vi "Command Voltages Check.vi"() -> ()   [LabVIEW 2009]
uses:
  lib/Apps/On Off Button.ctl
  lib/Calibration/Command Voltage Check Ramp States.ctl
  Test Utilities/DAQ Read Actions.ctl
  <vilib>/DAQmx/write.llb/DAQmx Write (Analog 1D DBL NChan 1Samp).vi
  C:/Program Files (x86)/National Instruments/LabVIEW 2009/resource/objmgr/daqmx.rc
panel:
  out "Cmd Volt Chk Ramp States":T1
  in  "Ramping":T2
  in  "Number of\nIntervals":i32
  in  "Half Period (msec)":i32
  in  "Peak Value":dbl
  in  "Offset":dbl
  out "Diffs":dbl[](array[numeric])=[-7.680882880270997, -8.566659800159199, -9.658116593296763, -9.594949810916727, -8.940447035067507, -8.192445315897492] format="%^#_10g"
  out "Write error out":errorcluster
  out "Monitor":dbl[](array[numeric])=[-7.680882880270997, -8.566659800159199, -9.658116593296763, -9.594949810916727, -8.940447035067507, -8.192445315897492] format="%^#_10g"
  out "Command \nVoltage":dbl[](array[numeric])=[-0.0, -0.0, -0.0, -0.0, -0.0, -0.0] format="%^#_10g"
  out "Control Voltage":dbl[](array[numeric])=[-0.0, -0.0, -0.0, -0.0, -0.0, -0.0]
  in  "Quit":bool
  in  "rate":dbl=100.0
  in  "samples per \nchannel":i32=30 caption="samples per channel"
  in  "Command Voltage Task":refnum<k21>="Command Voltage"
  in  "Monitor Task":refnum<k21>="All Readings"
  in  "Actuator":i32(listbox)
  out "Command \nVoltages":T3(graph)={"Average[0]"=-7.17251209904047, "Average[1]"=-8.19396103384171, "Average[2]"=-9.68369051887908, "Average[3]"=-9.45574535938537, "Average[4]"=-9.241187346298316, "Average[5]"=-8.612741694704903, "Average[6]"=0.0, "Average[7]"=0.0, "Average[8]"=0.0}
  out "Monitor":T3(graph)={"Average[0]"=-7.17251209904047, "Average[1]"=-8.19396103384171, "Average[2]"=-9.68369051887908, "Average[3]"=-9.45574535938537, "Average[4]"=-9.241187346298316, "Average[5]"=-8.612741694704903, "Average[6]"=0.0, "Average[7]"=0.0, "Average[8]"=0.0}
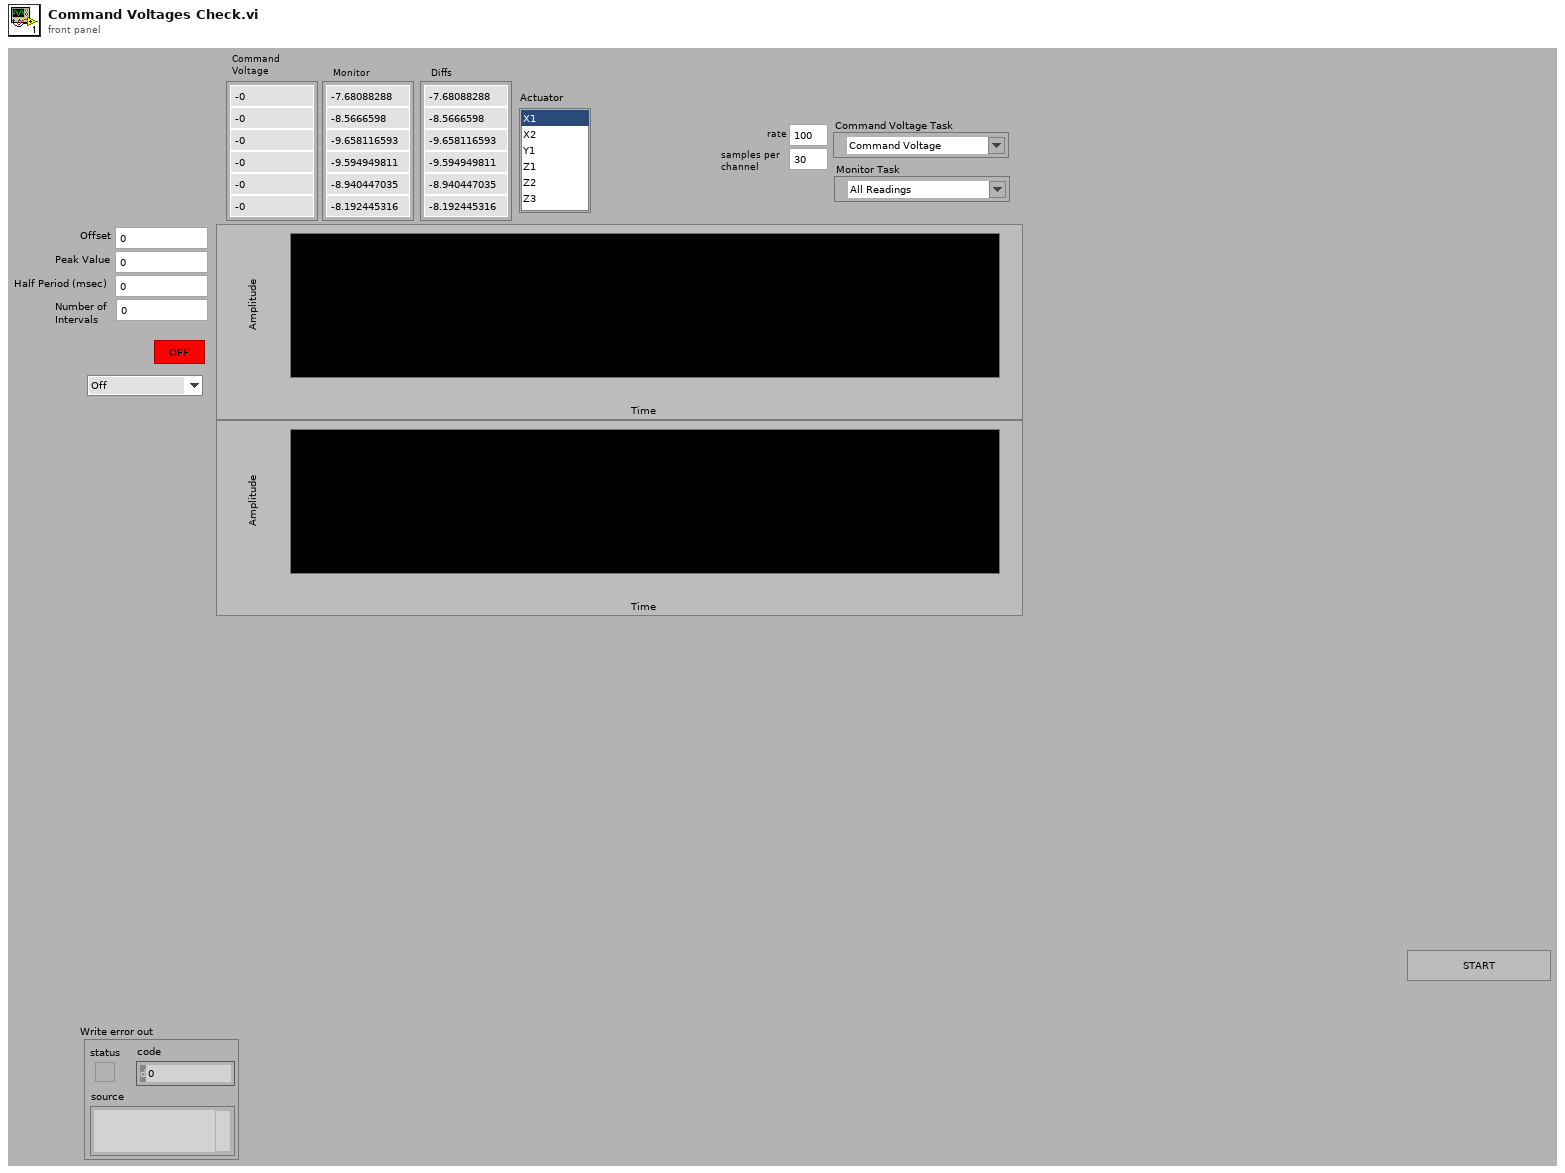
[diagram p1: front panel]
types:
  T1 = typedef "Command Voltage Check Ramp States.ctl" = enum16{"Off", "Start", "Ramp Up", "Ramp Down", "Stop"}
  T2 = typedef "On Off Button.ctl" = bool
  T3 = cluster{"Average[0]":dbl, "Average[1]":dbl, "Average[2]":dbl, "Average[3]":dbl, "Average[4]":dbl, "Average[5]":dbl, "Average[6]":dbl, "Average[7]":dbl, "Average[8]":dbl}
  T4 = typedef "DAQ Read Actions.ctl" = enum16{"Start", "Read", "Stop"}
  T5 = cluster{"Control Voltage[0]":dbl, "Control Voltage[1]":dbl, "Control Voltage[2]":dbl, "Control Voltage[3]":dbl, "Control Voltage[4]":dbl, "Control Voltage[5]":dbl, "Control Voltage[6]":dbl, "Control Voltage[7]":dbl, "Control Voltage[8]":dbl}
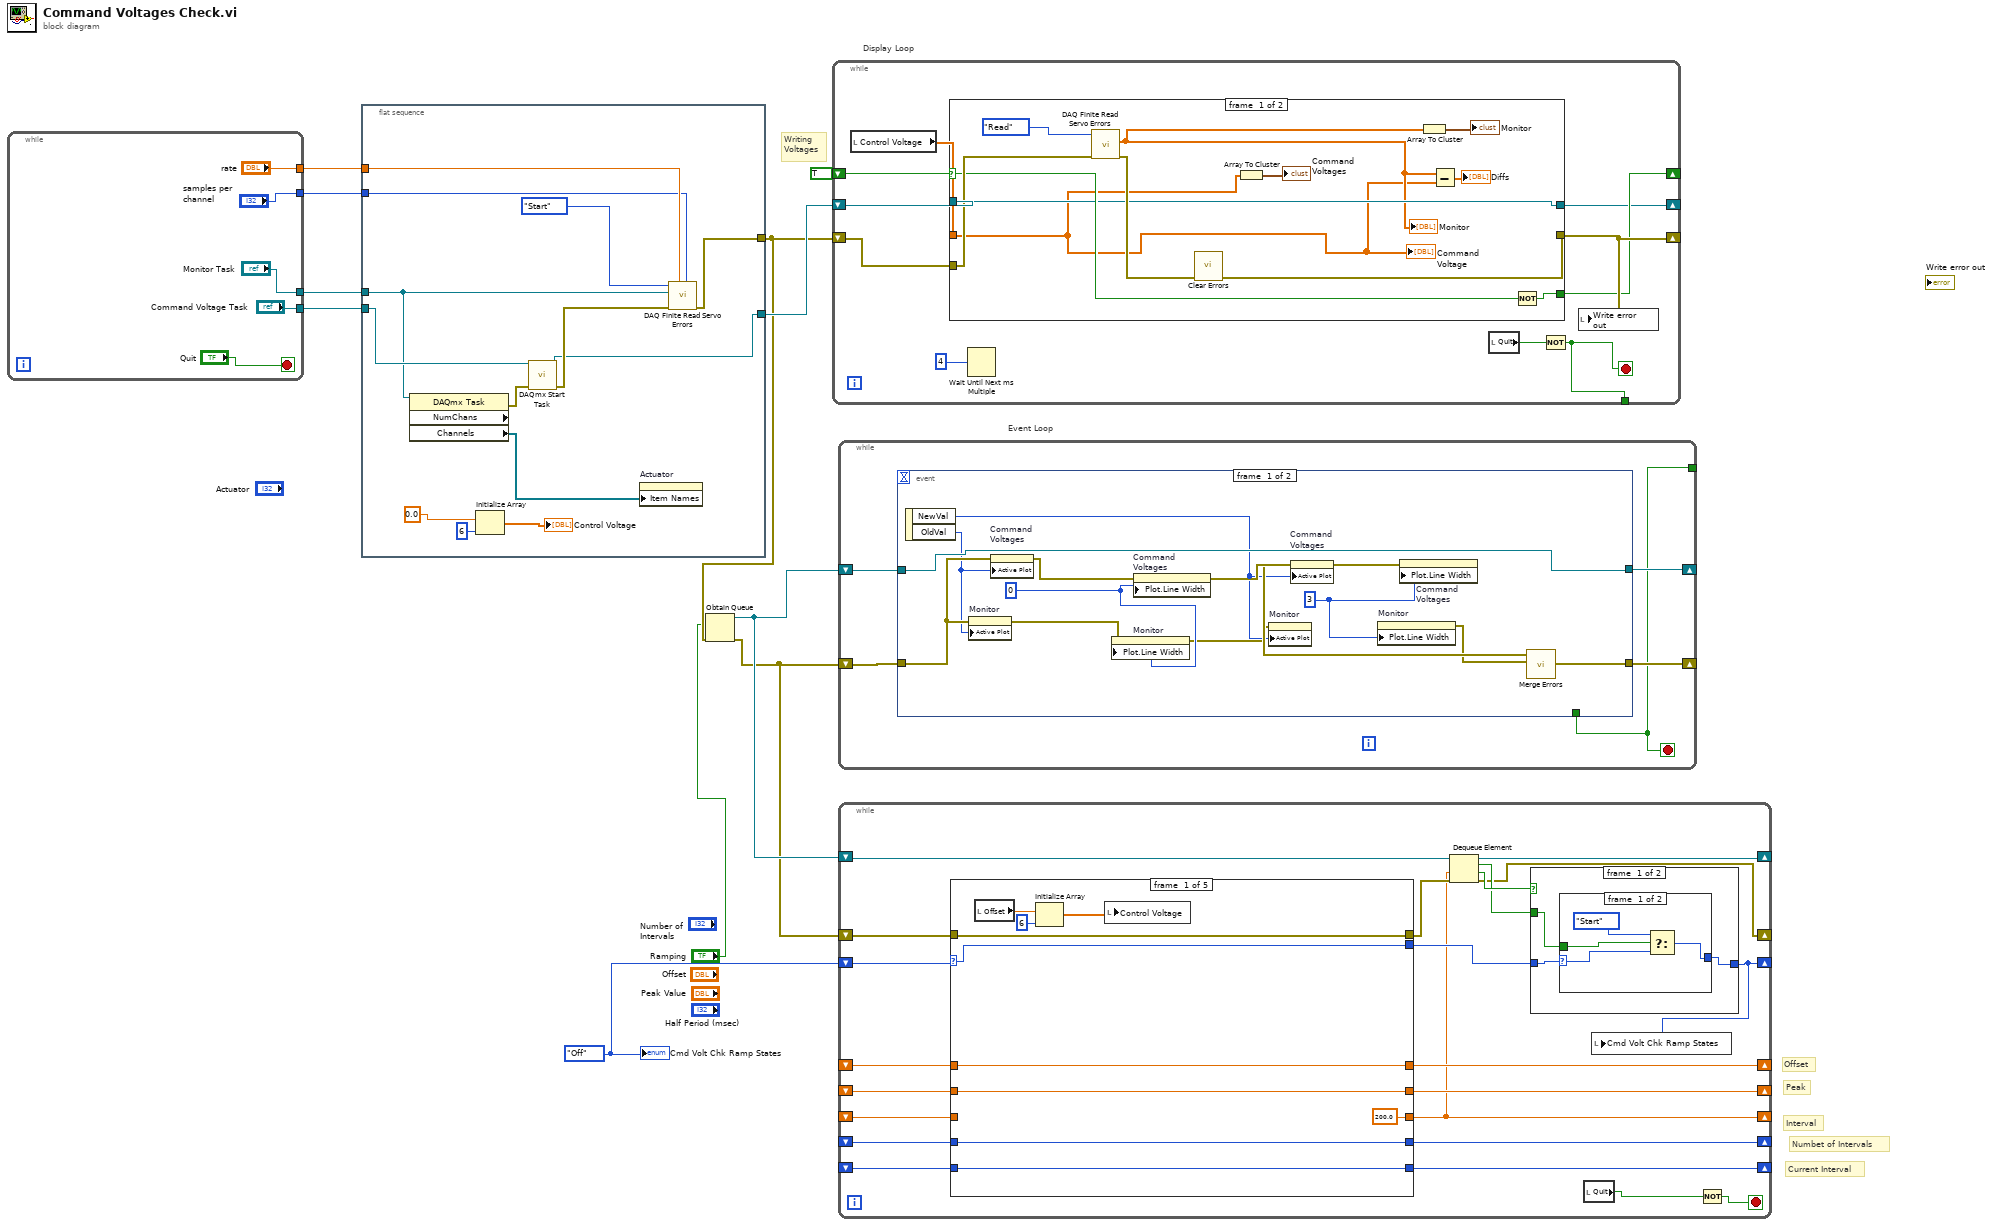
[diagram p0: block diagram]
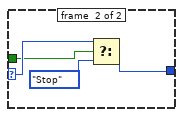
[diagram p2: hidden frame]
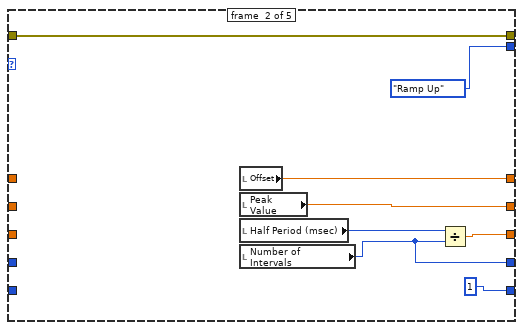
[diagram p4: hidden frame]
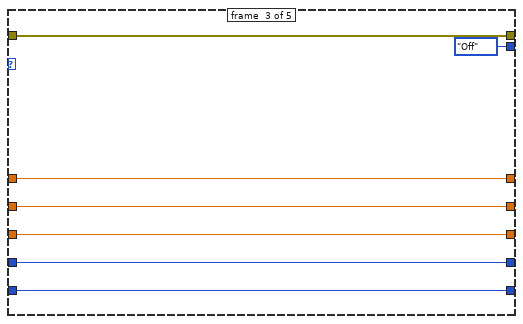
[diagram p5: hidden frame]
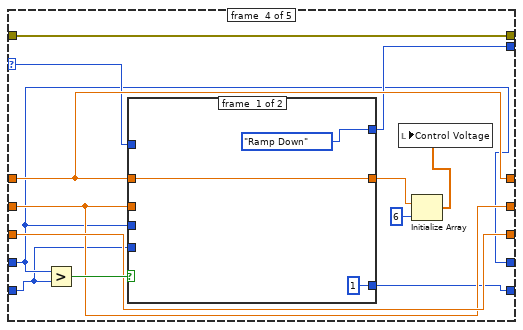
[diagram p6: hidden frame]
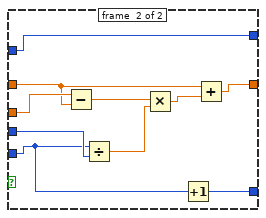
[diagram p7: hidden frame]
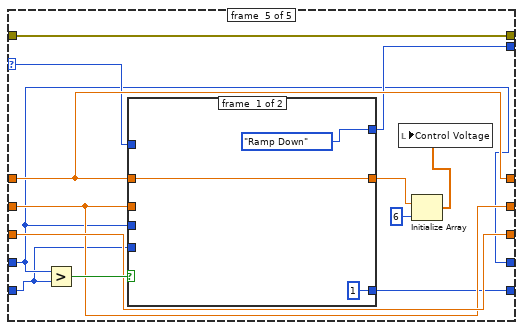
[diagram p8: hidden frame]
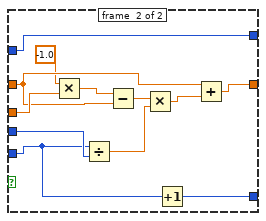
[diagram p9: hidden frame]
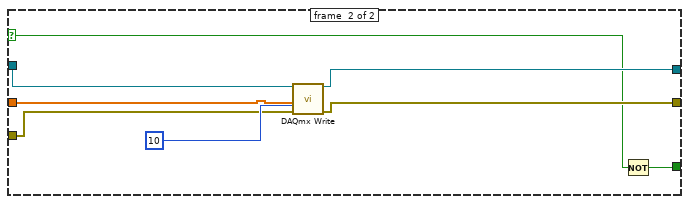
[diagram p10: hidden frame]
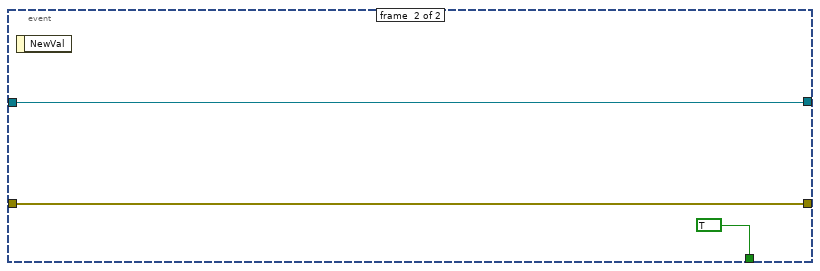
[diagram p11: hidden frame]
diagram:
  w5 = Command_Voltage_Check_Ramp_States."Off" ("Cmd Volt Chk Ramp States")
  # "Current Interval"
  # "Numbet of Intervals"
  # "Interval"
  # "Peak"
  # "Offset"
  # "Writing\nVoltages"
  n1 = while {
    tunnel: ["Command Voltage Task"] -> w11
    tunnel: ["Monitor Task"] -> w10
    tunnel: ["rate"] -> w9
    tunnel: ["samples per \nchannel"] -> w8
    stop <- "Quit" stop-if-true
  }
  n2 = flat-sequence {
    tunnel: w11 -> [w28]
    tunnel: w10 -> [w19]
    tunnel: w9 -> [w27]
    tunnel: w8 -> [w26]
    tunnel: [w21] -> w4
    tunnel: [w20] -> w7
    frame #0 {
      n3 = property class="DAQmx Task" props=["NumChans", "Channels"](reference=w19) -> (error out=w18:errorcluster, "Channels"=w17:refnum<k21>[])  [unwired: 1 in, 2 out]
      n4 = Initialize Array(0.0, 6 ("dimension size")) -> (→"Control Voltage":dbl[])
      n5 = call <vilib>:"DAQmx Start Task.vi"("task/channels in"=w28, "error in"=w18) -> ("task out"=w20:refnum<k21>, "error out"=w22:errorcluster)  [unwired: 12 out]
      n6 = property on="Actuator" class="LstBox (strict)"("Item Names"=w17) -> ()  [unwired: 2 in, 2 out]
      n7 = call "DAQ Finite Read Servo Errors.vi"("samples per channel"=w26, "rate"=w27, "error in"=w22, "task/channels in"=w19, "Action"=DAQ_Read_Actions."Start") -> ("error out"=w21:errorcluster)  [unwired: 6 out]
    }
  }
  n8 = Obtain Queue(element data type="Ramping", error in (no error)=w4) -> (queue out=w3:refnum<queue>, error out=w1:errorcluster)  [unwired: 3 in, 1 out]
  n9 = while "Display Loop" {
    shift-right: [w34] -> _
    shift-left: w4 -> [w35]
    tunnel: [w37] -> _
    shift-right: [w33] -> _
    shift-left: TRUE -> [w32]
    shift-right: [w30] -> _
    shift-left: w7 -> [w31]
    stop <- w37 stop-if-true
    n10 = local read "Control Voltage"() -> (w36:dbl[])
    n11 = case shown="False" w32 {
      selector: w32 -> [w45 w52]
      tunnel: w36 -> [w40 w55]
      tunnel: w35 -> [w48 w57]
      tunnel: [w46 w56] -> w34
      tunnel: [w44 w53] -> w33
      tunnel: w31 -> [w43 w58]
      tunnel: [w43 w54] -> w30
      frame #0 {
        n12 = call "DAQ Finite Read Servo Errors.vi"("error in"=w48, "Action"=DAQ_Read_Actions."Read") -> ("error out"=w47:errorcluster, "Average"=w41:dbl[])  [unwired: 3 in, 5 out]
        "Monitor" <- w41
        n13 = call <vilib>:"Clear Errors.vi"("error in (no error)"=w47) -> ("error out"=w46:errorcluster)  [unwired: 6 out]
        n14 = Array To Cluster(array=w40) -> (cluster=→"Command \nVoltages":T5)
        n15 = Array To Cluster(array=w41) -> (cluster=→"Monitor":T3)
        n16 = Subtract(x=w41, y=w40) -> (x-y=→"Diffs":dbl[])
        n17 = Not(x=w45) -> (.not. x?=w44:bool)
        "Command \nVoltage" <- w40
      }
      frame #1 {
        n18 = call-poly <vilib>:"DAQmx Write.vi"("task/channels in"=w58, "data"=w55, "timeout"=10, "error in"=w57) -> ("task out"=w54:refnum<k21>, "error out"=w56:errorcluster)  [unwired: 1 in, 9 out]
        n19 = Not(x=w52) -> (.not. x?=w53:bool)
      }
    }
    n20 = Wait Until Next ms Multiple(millisecond multiple=4) -> ()  [unwired: 1 out]
    n21 = local read "Quit"() -> (w38:bool)
    n22 = Not(x=w38) -> (.not. x?=w37:bool)
    n23 = local write "Write error out"(w34) -> ()
  }
  n24 = while "Event Loop" {
    tunnel: [w60] -> _
    shift-right: [w61] -> _
    shift-left: w1 -> [w63]
    shift-right: [w62] -> _
    shift-left: w3 -> [w64]
    stop <- w60 stop-if-true
    n25 = event shown="[1] \"Quit\": Value Change" {
      selector: _ -> [_ _]
      dyn-events: _ -> [_ _]
      timeout: _ -> [_ _]
      tunnel: w64 -> [w74 w79]
      tunnel: w63 -> [w73 w80]
      tunnel: [w74 w79] -> w62
      tunnel: [w66 w80] -> w61
      tunnel: [_ TRUE] -> w60
      event #0 {
        w67 = u8 3 ("Plot.Line Width")
        w71 = u8 0 ("Plot.Line Width")
        n26 = event-data() -> ("NewVal"=w68:i32, "OldVal"=w72:i32)  [unwired: 1 out]
        n27 = property on="Monitor" class="WFChart (strict)"(error in=w73, "Active Plot"=w72) -> (error out=w70:errorcluster)  [unwired: 1 in, 1 out]
        n28 = property on="Command \nVoltages" class="WFChart (strict)"(error in=w73, "Active Plot"=w72) -> (error out=w78:errorcluster)  [unwired: 1 in, 1 out]
        n29 = property on="Monitor" class="WFChart (strict)"(error in=w70, "Plot.Line Width"=w71) -> (error out=w69:errorcluster)  [unwired: 1 in, 1 out]
        n30 = property on="Command \nVoltages" class="WFChart (strict)"(error in=w78, "Plot.Line Width"=w71) -> (error out=w77:errorcluster)  [unwired: 1 in, 1 out]
        n31 = property on="Monitor" class="WFChart (strict)"(error in=w69, "Active Plot"=w68) -> ()  [unwired: 1 in, 2 out]
        n32 = property on="Command \nVoltages" class="WFChart (strict)"(error in=w77, "Active Plot"=w68) -> (error out=w76:errorcluster)  [unwired: 1 in, 1 out]
        n33 = property on="Monitor" class="WFChart (strict)"("Plot.Line Width"=w67) -> (error out=w65:errorcluster)  [unwired: 2 in, 1 out]
        n34 = property on="Command \nVoltages" class="WFChart (strict)"(error in=w76, "Plot.Line Width"=w67) -> (error out=w75:errorcluster)  [unwired: 1 in, 1 out]
        n35 = call <vilib>:"Merge Errors.vi"("error in 2 (no error)"=w65, "error in 1 (no error)"=w75) -> ("error out"=w66:errorcluster)  [unwired: 5 in]
      }
      event #1 {
        n36 = event-data() -> ()  [unwired: 2 out]
      }
    }
  }
  n37 = while {
    shift-right: [w85] -> _
    shift-left: w5 -> [w103]
    shift-right: [w96] -> _
    shift-left: w1 -> [w102]
    shift-right: [w95] -> _
    shift-left: w3 -> [w101]
    shift-right: [w84] -> _
    shift-left: _ -> [w88]
    shift-right: [w93] -> _
    shift-left: _ -> [w89]
    shift-right: [w94] -> _
    shift-left: _ -> [w90]
    shift-right: [w92] -> _
    shift-left: _ -> [w87]
    shift-right: [w91] -> _
    shift-left: _ -> [w86]
    stop <- w83 stop-if-true
    n38 = case shown="\"Stop\"" w103 {
      selector: w103 -> [w121 _ _ w145 w171]
      tunnel: w102 -> [w122 w126 w135 w153 w179]
      tunnel: [w122 w126 w135 w153 w179] -> w100
      tunnel: [w121 Command_Voltage_Check_Ramp_States."Ramp Up" ("Cmd Volt Chk Ramp States") Command_Voltage_Check_Ramp_States."Off" ("Cmd Volt Chk Ramp States") w144 w170] -> w97
      tunnel: [w120 w133 w140 w147 w173] -> w94
      tunnel: [w119 w132 w139 w146 w172] -> w93
      tunnel: [200.0 w130 w136 w151 w177] -> w84
      tunnel: [w117 w129 w138 w143 w169] -> w92
      tunnel: [w116 1 w137 w141 w167] -> w91
      tunnel: w90 -> [w120 _ w140 w147 w173]
      tunnel: w89 -> [w119 _ w139 w146 w172]
      tunnel: w88 -> [_ _ w136 w151 w177]
      tunnel: w87 -> [w117 _ w138 w143 w169]
      tunnel: w86 -> [w116 _ w137 w142 w168]
      frame #0 {
        n39 = local read "Offset"() -> (w125:dbl)
        n40 = Initialize Array(w125, 6 ("dimension size")) -> (w123:dbl[])
        n41 = local write "Control Voltage"(w123) -> ()
      }
      frame #1 {
        n42 = local read "Offset"() -> (w133:dbl)
        n43 = local read "Peak Value"() -> (w132:dbl)
        n44 = local read "Half Period (msec)"() -> (w131:i32)
        n45 = local read "Number of\nIntervals"() -> (w129:i32)
        n46 = Divide(x=w131, y=w129) -> (x/y=w130:dbl)
      }
      frame #2 {
      }
      frame #3 {
        n47 = Greater?(x=w143, y=w142) -> (0:w152:bool)
        n48 = case shown="False" w152 {
          tunnel: w146 -> [_ w162]
          tunnel: w147 -> [w156 w161]
          tunnel: [w156 w159] -> w149
          tunnel: w145 -> [_ w166]
          tunnel: [Command_Voltage_Check_Ramp_States."Ramp Down" ("Cmd Volt Chk Ramp States") w166] -> w144
          tunnel: w143 -> [_ w165]
          tunnel: w142 -> [_ w158]
          tunnel: [1 w157] -> w141
          frame #0 {
          }
          frame #1 {
            n49 = Subtract(x=w162, y=w161) -> (x-y=w164:dbl)
            n50 = Divide(x=w158, y=w165) -> (x/y=w163:dbl)
            n51 = Multiply(x=w164, y=w163) -> (x*y=w160:dbl)
            n52 = Increment(x=w158) -> (x+1=w157:i32)
            n53 = Add(x=w161, y=w160) -> (x+y=w159:dbl)
          }
        }
        n54 = Initialize Array(w149, 6 ("dimension size")) -> (w148:dbl[])
        n55 = local write "Control Voltage"(w148) -> ()
      }
      frame #4 {
        n56 = Greater?(x=w169, y=w168) -> (0:w178:bool)
        n57 = case shown="False" w178 {
          tunnel: w172 -> [_ w190]
          tunnel: w173 -> [w182 w189]
          tunnel: [w182 w187] -> w175
          tunnel: w171 -> [_ w194]
          tunnel: [Command_Voltage_Check_Ramp_States."Ramp Down" ("Cmd Volt Chk Ramp States") w194] -> w170
          tunnel: w169 -> [_ w193]
          tunnel: w168 -> [_ w184]
          tunnel: [1 w183] -> w167
          frame #0 {
          }
          frame #1 {
            n58 = Multiply(x=-1.0, y=w190) -> (x*y=w186:dbl)
            n59 = Divide(x=w184, y=w193) -> (x/y=w191:dbl)
            n60 = Subtract(x=w186, y=w189) -> (x-y=w192:dbl)
            n61 = Multiply(x=w192, y=w191) -> (x*y=w188:dbl)
            n62 = Increment(x=w184) -> (x+1=w183:i32)
            n63 = Add(x=w189, y=w188) -> (x+y=w187:dbl)
          }
        }
        n64 = Initialize Array(w175, 6 ("dimension size")) -> (w174:dbl[])
        n65 = local write "Control Voltage"(w174) -> ()
      }
    }
    n66 = Dequeue Element(queue=w101, timeout in ms (-1)=w84, error in (no error)=w100) -> (queue out=w95:refnum<queue>, element=w98:T2, timed out?=w99:bool, error out=w96:errorcluster)
    n67 = case shown="False" w99 {
      tunnel: w98 -> [w105 _]
      tunnel: w97 -> [w106 w115]
      tunnel: [w104 w115] -> w85
      frame #0 {
        n68 = case shown="\"Start\", Default" w106 {
          selector: w106 -> [w109 w114]
          tunnel: w105 -> [w110 w113]
          tunnel: [w108 w111] -> w104
          frame #0 {
            n69 = Select(t=Command_Voltage_Check_Ramp_States."Start", s=w110, f=w109) -> (s? t:f=w108:T1)
          }
          frame #1 {
            n70 = Select(t=w114, s=w113, f=Command_Voltage_Check_Ramp_States."Stop") -> (s? t:f=w111:T1)
          }
        }
      }
      frame #1 {
      }
    }
    n71 = local read "Quit"() -> (w82:bool)
    n72 = local write "Cmd Volt Chk Ramp States"(w85) -> ()
    n73 = Not(x=w82) -> (.not. x?=w83:bool)
  }
  "Cmd Volt Chk Ramp States" <- w5
